vi "CurveFit2.vi"(8 "Right Motor Power":i8, 11 "Left Motor Power":i8) -> (0 "Right Motor Output":i8, 3 "Left Motor Output":i8)   [LabVIEW 2012]
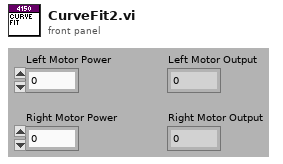
[diagram p1: front panel]
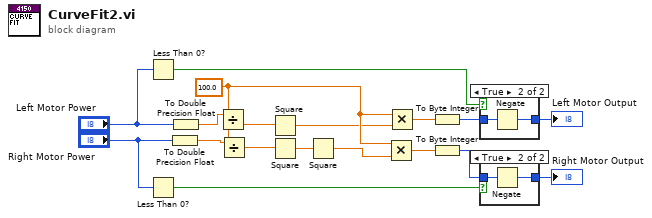
[diagram p0: block diagram]
diagram:
  w10 = 100.0
  n1 = Less Than 0?(x="Left Motor Power") -> (x < 0?=w14:bool)
  n2 = Less Than 0?(x="Right Motor Power") -> (x < 0?=w18:bool)
  n3 = To Double Precision Float(number="Right Motor Power") -> (double precision float=w5:dbl)
  n4 = To Double Precision Float(number="Left Motor Power") -> (double precision float=w4:dbl)
  n5 = Divide(x=w4, y=w10) -> (x/y=w2:dbl)
  n6 = Divide(x=w5, y=w10) -> (x/y=w3:dbl)
  n7 = Square(x=w2) -> (x^2=w6:dbl)
  n8 = Square(x=w3) -> (x^2=w7:dbl)
  n9 = Square(x=w7) -> (x^2=w1:dbl)
  n10 = Multiply(x=w10, y=w1) -> (x*y=w8:dbl)
  n11 = Multiply(x=w10, y=w6) -> (x*y=w9:dbl)
  n12 = To Byte Integer(number=w9) -> (8bit integer=w13:i8)
  n13 = To Byte Integer(number=w8) -> (8bit integer=w16:i8)
  n14 = case shown="True" w14 {
    tunnel: [w19 w20] -> w15
    tunnel: w13 -> [w19 w21]
    frame False {
    }
    frame True {
      n15 = Negate(x=w21) -> (-x=w20:i8)
    }
  }
  "Left Motor Output" <- w15
  n16 = case shown="True" w18 {
    tunnel: [w22 w23] -> w17
    tunnel: w16 -> [w22 w24]
    frame False {
    }
    frame True {
      n17 = Negate(x=w24) -> (-x=w23:i8)
    }
  }
  "Right Motor Output" <- w17
